vi "5_Dice(170382,170307).vi"() -> ()   [LabVIEW 2015]
panel:
  out "Win Indicator":bool
  out "Dice rolls":dbl
  out "No. of wins":u64
  out "D2":dbl
  out "D1":dbl
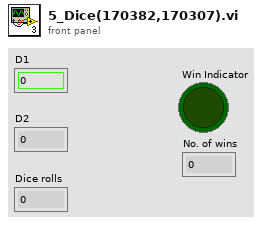
[diagram p1: front panel]
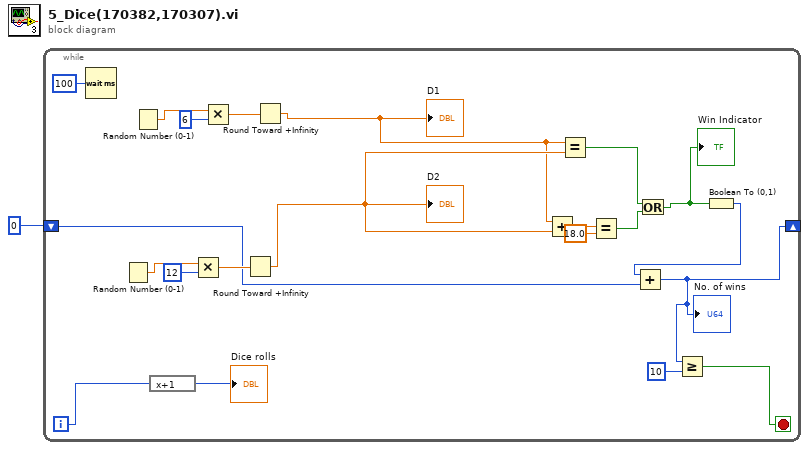
[diagram p0: block diagram]
diagram:
  n1 = while {
    shift-right: [w8] -> _
    shift-left: 0 -> [w10]
    i -> [w4]
    stop <- w6 stop-if-true
    n2 = Wait (ms)(milliseconds to wait=u32 100) -> ()  [unwired: 1 out]
    n3 = Random Number (0-1)() -> (number: 0 to 1=w19:dbl)
    n4 = Random Number (0-1)() -> (number: 0 to 1=w20:dbl)
    n5 = expression code="x+1"(w4) -> (→"Dice rolls":i32)
    n6 = Multiply(x=w19, y=i64 12) -> (x*y=w17:dbl)
    n7 = Multiply(x=w20, y=i64 6) -> (x*y=w22:dbl)
    n8 = Round Toward +Infinity(x=w17) -> (ceil(x): smallest int >= x=w15:dbl)
    "D2" <- w15
    n9 = Round Toward +Infinity(x=w22) -> (ceil(x): smallest int >= x=w14:dbl)
    "D1" <- w14
    n10 = Add(x=w14, y=w15) -> (x+y=w13:dbl)
    n11 = Equal?(x=w14, y=w15) -> (x = y?=w16:bool)
    n12 = Equal?(x=w13, y=18.0) -> (x = y?=w11:bool)
    n13 = Or(x=w16, y=w11) -> (x .or. y?=w3:bool)
    "Win Indicator" <- w3
    n14 = Boolean To (0,1)(Boolean=w3) -> (0, 1=w9:i16)
    n15 = Add(x=w9, y=w10) -> (x+y=w8:i32)
    "No. of wins" <- w8
    n16 = Greater Or Equal?(x=w8, y=10) -> (x >= y?=w6:bool)
  }
